vi "nanocal -- nuclear schottky fit V8.vi"() -> ()   [LabVIEW 2021] (continued)
\"mm1\" -> 0.000000000000   ,  \"mm2\" -> 0.000000000000   ,  \"mm3\" -> 0.000000000000   ,  \"T\" -> 0.300000000000   ,  \"B\" -> 2.000000000000   ,  \"θ\" -> 90.000000000000   ,  \"Reoff\" -> 0.000000000000   ,  \"Imoff\" -> 0.000000000000   ,  \"στ1\" -> 0.000000000000   ,  \"στS\" -> 0.000000000000   ,  \"στN\" -> 0.000000000000   ,  \"τ11 \" -> 0.000000000000   ,  \"τ12\" -> 0.000000000000   ,  \"τ22\" -> 0.000000000000   ,  \"τN1\" -> 0.000000000000   ,  \"τN2\" -> 0.000000000000   ,  \"σηlogτ1 \" -> 0.000000000000   ,  \"σηlogτS\" -> 0.000000000000   ,  \"σηlogτN\" -> 0.000000000000   ,  \"σlogτ1\" -> 0.000000000000   ,  \"σlogτS\" -> 0.000000000000   ,  \"σlogτN\" -> 0.000000000000   ,  \"σητ1\" -> 0.000000000000   ,  \"σητS \" -> 0.000000000000   ,  \"σητN\" -> 0.000000000000    |>   , \r\"IDS0584_220608_RAW_cal__ref_\" ->   <|    \"ζ\" -> 0.081243214747   ,  \"τ1\" -> 0.037135443189   ,  \"τS\" -> 0.014363776862   ,  \"τN\" -> 0.000724531165   ,  \"τC\" -> 0.001657389357   ,  \"κ0\" -> 0.000000001966   ,  \"mm1\" -> 0.000113270602   ,  \"mm2\" -> 0.016452146337   ,  \"mm3\" -> 0.038541546284   ,  \"T\" -> 0.360000000000   ,  \"B\" -> 2.000000000000   ,  \"θ\" -> 90.000000000000   ,  \"Reoff\" -> 0.000000000000   ,  \"Imoff\" -> 0.000000000000   ,  \"στ1\" -> 0.000570634052   ,  \"στS\" -> 0.000001716733   ,  \"στN\" -> 0.000008284109   ,  \"τ11 \" -> 0.000000000000   ,  \"τ12\" -> 0.000000000000   ,  \"τ22\" -> 0.000000000000   ,  \"τN1\" -> 0.000000000000   ,  \"τN2\" -> 0.000000000000   ,  \"σηlogτ1 \" -> 0.079922172346   ,  \"σηlogτS\" -> 0.000048378934   ,  \"σηlogτN\" -> 0.121081817682   ,  \"σlogτ1\" -> 0.015366291700   ,  \"σlogτS\" -> 0.000119518229   ,  \"σlogτN\" -> 0.011433750926   ,  \"σητ1\" -> 0.002967945291   ,  \"σητS \" -> 0.000000694904   ,  \"σητN\" -> 0.000087727550    |>   , \r\"IDS0584_220608_RAW_cal__sam_\" ->   <|    \"ζ\" -> 0.000000000000   ,  \"τ1\" -> 0.000000000000   ,  \"τS\" -> 0.000000000000   ,  \"τN\" -> 0.000000000000   ,  \"τC\" -> 0.000000000000   ,  \"κ0\" -> 0.000000000000   ,  \"mm1\" -> 0.000000000000   ,  \"mm2\" -> 0.000000000000   ,  \"mm3\" -> 0.000000000000   ,  \"T\" -> 0.360000000000   ,  \"B\" -> 2.000000000000   ,  \"θ\" -> 90.000000000000   ,  \"Reoff\" -> 0.000000000000   ,  \"Imoff\" -> 0.000000000000   ,  \"στ1\" -> 0.000000000000   ,  \"στS\" -> 0.000000000000   ,  \"στN\" -> 0.000000000000   ,  \"τ11 \" -> 0.000000000000   ,  \"τ12\" -> 0.000000000000   ,  \"τ22\" -> 0.000000000000   ,  \"τN1\" -> 0.000000000000   ,  \"τN2\" -> 0.000000000000   ,  \"σηlogτ1 \" -> 0.000000000000   ,  \"σηlogτS\" -> 0.000000000000   ,  \"σηlogτN\" -> 0.000000000000   ,  \"σlogτ1\" -> 0.000000000000   ,  \"σlogτS\" -> 0.000000000000   ,  \"σlogτN\" -> 0.000000000000   ,  \"σητ1\" -> 0.000000000000   ,  \"σητS \" -> 0.000000000000   ,  \"σητN\" -> 0.000000000000    |>   , \r\"IDS0585_220608_RAW_cal__ref_\" ->   <|    \"ζ\" -> 0.062678864922   ,  \"τ1\" -> 0.031193965489   ,  \"τS\" -> 0.014071158439   ,  \"τN\" -> 0.000589761795   ,  \"τC\" -> 0.002071432088   ,  \"κ0\" -> 0.000000002372   ,  \"mm1\" -> 0.000107994659   ,  \"mm2\" -> 0.016236809619   ,  \"mm3\" -> 0.032500443372   ,  \"T\" -> 0.420000000000   ,  \"B\" -> 2.000000000000   ,  \"θ\" -> 90.000000000000   ,  \"Reoff\" -> 0.000000000000   ,  \"Imoff\" -> 0.000000000000   ,  \"στ1\" -> 0.000397411460   ,  \"στS\" -> 0.000001349493   ,  \"στN\" -> 0.000005324437   ,  \"τ11 \" -> 0.000000000000   ,  \"τ12\" -> 0.000000000000   ,  \"τ22\" -> 0.000000000000   ,  \"τN1\" -> 0.000000000000   ,  \"τN2\" -> 0.000000000000   ,  \"σηlogτ1 \" -> 0.084702441661   ,  \"σηlogτS\" -> 0.000054291410   ,  \"σηlogτN\" -> 0.122395661985   ,  \"σlogτ1\" -> 0.012740010877   ,  \"σlogτS\" -> 0.000095904870   ,  \"σlogτN\" -> 0.009028114419   ,  \"σητ1\" -> 0.002642205042   ,  \"σητS \" -> 0.000000763943   ,  \"σητN\" -> 0.000072184285    |>   , \r\"IDS0585_220608_RAW_cal__sam_\" ->   <|    \"ζ\" -> 0.000000000000   ,  \"τ1\" -> 0.000000000000   ,  \"τS\" -> 0.000000000000   ,  \"τN\" -> 0.000000000000   ,  \"τC\" -> 0.000000000000   ,  \"κ0\" -> 0.000000000000   ,  \"mm1\" -> 0.000000000000   ,  \"mm2\" -> 0.000000000000   ,  \"mm3\" -> 0.000000000000   ,  \"T\" -> 0.420000000000   ,  \"B\" -> 2.000000000000   ,  \"θ\" -> 90.000000000000   ,  \"Reoff\" -> 0.000000000000   ,  \"Imoff\" -> 0.000000000000   ,  \"στ1\" -> 0.000000000000   ,  \"στS\" -> 0.000000000000   ,  \"στN\" -> 0.000000000000   ,  \"τ11 \" -> 0.000000000000   ,  \"τ12\" -> 0.000000000000   ,  \"τ22\" -> 0.000000000000   ,  \"τN1\" -> 0.000000000000   ,  \"τN2\" -> 0.000000000000   ,  \"σηlogτ1 \" -> 0.000000000000   ,  \"σηlogτS\" -> 0.000000000000   ,  \"σηlogτN\" -> 0.000000000000   ,  \"σlogτ1\" -> 0.000000000000   ,  \"σlogτS\" -> 0.000000000000   ,  \"σlogτN\" -> 0.000000000000   ,  \"σητ1\" -> 0.000000000000   ,  \"σητS \" -> 0.000000000000   ,  \"σητN\" -> 0.000000000000    |>   , \r\"IDS0586_220608_RAW_cal__ref_\" ->   <|    \"ζ\" -> 0.045613371440   ,  \"τ1\" -> 0.021724714281   ,  \"τS\" -> 0.014809258132   ,  \"τN\" -> 0.000242258752   ,  \"τC\" -> 0.002279252740   ,  \"κ0\" -> 0.000000003040   ,  \"mm1\" -> 0.000087097961   ,  \"mm2\" -> 0.016810935074   ,  \"mm3\" -> 0.022844001300   ,  \"T\" -> 0.520000000000   ,  \"B\" -> 2.000000000000   ,  \"θ\" -> 90.000000000000   ,  \"Reoff\" -> 0.000000000000   ,  \"Imoff\" -> 0.000000000000   ,  \"στ1\" -> 0.000379951004   ,  \"στS\" -> 0.000001062979   ,  \"στN\" -> 0.000002619514   ,  \"τ11 \" -> 0.000000000000   ,  \"τ12\" -> 0.000000000000   ,  \"τ22\" -> 0.000000000000   ,  \"τN1\" -> 0.000000000000   ,  \"τN2\" -> 0.000000000000   ,  \"σηlogτ1 \" -> 0.100214341065   ,  \"σηlogτS\" -> 0.000043367653   ,  \"σηlogτN\" -> 0.126292121784   ,  \"σlogτ1\" -> 0.017489344108   ,  \"σlogτS\" -> 0.000071778006   ,  \"σlogτN\" -> 0.010812876419   ,  \"σητ1\" -> 0.002177127926   ,  \"σητS \" -> 0.000000642243   ,  \"σητN\" -> 0.000030595372    |>   , \r\"IDS0586_220608_RAW_cal__sam_\" ->   <|    \"ζ\" -> 0.000000000000   ,  \"τ1\" -> 0.000000000000   ,  \"τS\" -> 0.000000000000   ,  \"τN\" -> 0.000000000000   ,  \"τC\" -> 0.000000000000   ,  \"κ0\" -> 0.000000000000   ,  \"mm1\" -> 0.000000000000   ,  \"mm2\" -> 0.000000000000   ,  \"mm3\" -> 0.000000000000   ,  \"T\" -> 0.520000000000   ,  \"B\" -> 2.000000000000   ,  \"θ\" -> 90.000000000000   ,  \"Reoff\" -> 0.000000000000   ,  \"Imoff\" -> 0.000000000000   ,  \"στ1\" -> 0.000000000000   ,  \"στS\" -> 0.000000000000   ,  \"στN\" -> 0.000000000000   ,  \"τ11 \" -> 0.000000000000   ,  \"τ12\" -> 0.000000000000   ,  \"τ22\" -> 0.000000000000   ,  \"τN1\" -> 0.000000000000   ,  \"τN2\" -> 0.000000000000   ,  \"σηlogτ1 \" -> 0.000000000000   ,  \"σηlogτS\" -> 0.000000000000   ,  \"σηlogτN\" -> 0.000000000000   ,  \"σlogτ1\" -> 0.000000000000   ,  \"σlogτS\" -> 0.000000000000   ,  \"σlogτN\" -> 0.000000000000   ,  \"σητ1\" -> 0.000000000000   ,  \"σητS \" -> 0.000000000000   ,  \"σητN\" -> 0.000000000000    |>   , \r\"IDS0587_220608_RAW_cal__ref_\" ->   <|    \"ζ\" -> 0.037305312817   ,  \"τ1\" -> 0.022015385532   ,  \"τS\" -> 0.015983002513   ,  \"τN\" -> 0.000140757523   ,  \"τC\" -> 0.002926821930   ,  \"κ0\" -> 0.000000003719   ,  \"mm1\" -> 0.000089879141   ,  \"mm2\" -> 0.018616997914   ,  \"mm3\" -> 0.022960592355   ,  \"T\" -> 0.620000000000   ,  \"B\" -> 2.000000000000   ,  \"θ\" -> 90.000000000000   ,  \"Reoff\" -> 0.000000000000   ,  \"Imoff\" -> 0.000000000000   ,  \"στ1\" -> 0.001387023615   ,  \"στS\" -> 0.000002362873   ,  \"στN\" -> 0.000005327242   ,  \"τ11 \" -> 0.000000000000   ,  \"τ12\" -> 0.000000000000   ,  \"τ22\" -> 0.000000000000   ,  \"τN1\" -> 0.000000000000   ,  \"τN2\" -> 0.000000000000   ,  \"σηlogτ1 \" -> 0.104062754618   ,  \"σηlogτS\" -> 0.000026827334   ,  \"σηlogτN\" -> 0.127171087311   ,  \"σlogτ1\" -> 0.063002467668   ,  \"σlogτS\" -> 0.000147836639   ,  \"σlogτN\" -> 0.037846942559   ,  \"σητ1\" -> 0.002290981662   ,  \"σητS \" -> 0.000000428781   ,  \"σητN\" -> 0.000017900287    |>   , \r\"IDS0587_220608_RAW_cal__sam_\" ->   <|    \"ζ\" -> 0.000000000000   ,  \"τ1\" -> 0.000000000000   ,  \"τS\" -> 0.000000000000   ,  \"τN\" -> 0.000000000000   ,  \"τC\" -> 0.000000000000   ,  \"κ0\" -> 0.000000000000   ,  \"mm1\" -> 0.000000000000   ,  \"mm2\" -> 0.000000000000   ,  \"mm3\" -> 0.000000000000   ,  \"T\" -> 0.620000000000   ,  \"B\" -> 2.000000000000   ,  \"θ\" -> 90.000000000000   ,  \"Reoff\" -> 0.000000000000   ,  \"Imoff\" -> 0.000000000000   ,  \"στ1\" -> 0.000000000000   ,  \"στS\" -> 0.000000000000   ,  \"στN\" -> 0.000000000000   ,  \"τ11 \" -> 0.000000000000   ,  \"τ12\" -> 0.000000000000   ,  \"τ22\" -> 0.000000000000   ,  \"τN1\" -> 0.000000000000   ,  \"τN2\" -> 0.000000000000   ,  \"σηlogτ1 \" -> 0.000000000000   ,  \"σηlogτS\" -> 0.000000000000   ,  \"σηlogτN\" -> 0.000000000000   ,  \"σlogτ1\" -> 0.000000000000   ,  \"σlogτS\" -> 0.000000000000   ,  \"σlogτN\" -> 0.000000000000   ,  \"σητ1\" -> 0.000000000000   ,  \"σητS \" -> 0.000000000000   ,  \"σητN\" -> 0.000000000000    |>   , \r\"IDS0588_220608_RAW_cal__ref_\" ->   <|    \"ζ\" -> 0.025909739103   ,  \"τ1\" -> 0.011339568662   ,  \"τS\" -> 0.019465034891   ,  \"τN\" -> 0.000064248096   ,  \"τC\" -> 0.003634951458   ,  \"κ0\" -> 0.000000005097   ,  \"mm1\" -> 0.000077921965   ,  \"mm2\" -> 0.011278943418   ,  \"mm3\" -> 0.023652936351   ,  \"T\" -> 0.820000000000   ,  \"B\" -> 2.000000000000   ,  \"θ\" -> 90.000000000000   ,  \"Reoff\" -> 0.000000000000   ,  \"Imoff\" -> 0.000000000000   ,  \"στ1\" -> 0.000804918682   ,  \"στS\" -> 0.000001968832   ,  \"στN\" -> 0.000002244062   ,  \"τ11 \" -> 0.000000000000   ,  \"τ12\" -> 0.000000000000   ,  \"τ22\" -> 0.000000000000   ,  \"τN1\" -> 0.000000000000   ,  \"τN2\" -> 0.000000000000   ,  \"σηlogτ1 \" -> 0.166612292303   ,  \"σηlogτS\" -> 0.000038744835   ,  \"σηlogτN\" -> 0.138837522658   ,  \"σlogτ1\" -> 0.070983183376   ,  \"σlogτS\" -> 0.000101147100   ,  \"σlogτN\" -> 0.034928067640   ,  \"σητ1\" -> 0.001889311528   ,  \"σητS \" -> 0.000000754170   ,  \"σητN\" -> 0.000008920046    |>   , \r\"IDS0588_220608_RAW_cal__sam_\" ->   <|    \"ζ\" -> 0.000000000000   ,  \"τ1\" -> 0.000000000000   ,  \"τS\" -> 0.000000000000   ,  \"τN\" -> 0.000000000000   ,  \"τC\" -> 0.000000000000   ,  \"κ0\" -> 0.000000000000   ,  \"mm1\" -> 0.000000000000   ,  \"mm2\" -> 0.000000000000   ,  \"mm3\" -> 0.000000000000   ,  \"T\" -> 0.820000000000   ,  \"B\" -> 2.000000000000   ,  \"θ\" -> 90.000000000000   ,  \"Reoff\" -> 0.000000000000   ,  \"Imoff\" -> 0.000000000000   ,  \"στ1\" -> 0.000000000000   ,  \"στS\" -> 0.000000000000   ,  \"στN\" -> 0.000000000000   ,  \"τ11 \" -> 0.000000000000   ,  \"τ12\" -> 0.000000000000   ,  \"τ22\" -> 0.000000000000   ,  \"τN1\" -> 0.000000000000   ,  \"τN2\" -> 0.000000000000   ,  \"σηlogτ1 \" -> 0.000000000000   ,  \"σηlogτS\" -> 0.000000000000   ,  \"σηlogτN\" -> 0.000000000000   ,  \"σlogτ1\" -> 0.000000000000   ,  \"σlogτS\" -> 0.000000000000   ,  \"σlogτN\" -> 0.000000000000   ,  \"σητ1\" -> 0.000000000000   ,  \"σητS \" -> 0.000000000000   ,  \"σητN\" -> 0.000000000000    |>   , \r\"IDS0589_220608_RAW_cal__ref_\" ->   <|    \"ζ\" -> 0.019947361770   ,  \"τ1\" -> 0.011361864478   ,  \"τS\" -> 0.027583078448   ,  \"τN\" -> 0.000020419433   ,  \"τC\" -> 0.003703000671   ,  \"κ0\" -> 0.000000007195   ,  \"mm1\" -> 0.000064126126   ,  \"mm2\" -> 0.011350297657   ,  \"mm3\" -> 0.031804556205   ,  \"T\" -> 1.120000000000   ,  \"B\" -> 2.000000000000   ,  \"θ\" -> 90.000000000000   ,  \"Reoff\" -> 0.000000000000   ,  \"Imoff\" -> 0.000000000000   ,  \"στ1\" -> 0.003857512169   ,  \"στS\" -> 0.000003346779   ,  \"στN\" -> 0.000003441616   ,  \"τ11 \" -> 0.000000000000   ,  \"τ12\" -> 0.000000000000   ,  \"τ22\" -> 0.000000000000   ,  \"τN1\" -> 0.000000000000   ,  \"τN2\" -> 0.000000000000   ,  \"σηlogτ1 \" -> 0.199481573795   ,  \"σηlogτS\" -> 0.000012934123   ,  \"σηlogτN\" -> 0.143434929162   ,  \"σlogτ1\" -> 0.339514009879   ,  \"σlogτS\" -> 0.000121334492   ,  \"σlogτN\" -> 0.168546132727   ,  \"σητ1\" -> 0.002266482607   ,  \"σητS \" -> 0.000000356763   ,  \"σητN\" -> 0.000002928860    |>   , \r\"IDS0589_220608_RAW_cal__sam_\" ->   <|    \"ζ\" -> 0.000000000000   ,  \"τ1\" -> 0.000000000000   ,  \"τS\" -> 0.000000000000   ,  \"τN\" -> 0.000000000000   ,  \"τC\" -> 0.000000000000   ,  \"κ0\" -> 0.000000000000   ,  \"mm1\" -> 0.000000000000   ,  \"mm2\" -> 0.000000000000   ,  \"mm3\" -> 0.000000000000   ,  \"T\" -> 1.120000000000   ,  \"B\" -> 2.000000000000   ,  \"θ\" -> 90.000000000000   ,  \"Reoff\" -> 0.000000000000   ,  \"Imoff\" -> 0.000000000000   ,  \"στ1\" -> 0.000000000000   ,  \"στS\" -> 0.000000000000   ,  \"στN\" -> 0.000000000000   ,  \"τ11 \" -> 0.000000000000   ,  \"τ12\" -> 0.000000000000   ,  \"τ22\" -> 0.000000000000   ,  \"τN1\" -> 0.000000000000   ,  \"τN2\" -> 0.000000000000   ,  \"σηlogτ1 \" -> 0.000000000000   ,  \"σηlogτS\" -> 0.000000000000   ,  \"σηlogτN\" -> 0.000000000000   ,  \"σlogτ1\" -> 0.000000000000   ,  \"σlogτS\" -> 0.000000000000   ,  \"σlogτN\" -> 0.000000000000   ,  \"σητ1\" -> 0.000000000000   ,  \"σητS \" -> 0.000000000000   ,  \"σητN\" -> 0.000000000000    |>   , \r\"IDS0590_220608_RAW_cal__ref_\" ->   <|    \"ζ\" -> 0.015986824181   ,  \"τ1\" -> 0.008744331225   ,  \"τS\" -> 0.042647705878   ,  \"τN\" -> 0.000007777315   ,  \"τC\" -> 0.003875042779   ,  \"κ0\" -> 0.000000010497   ,  \"mm1\" -> 0.000056035896   ,  \"mm2\" -> 0.008742533558   ,  \"mm3\" -> 0.047158213453   ,  \"T\" -> 1.600000000000   ,  \"B\" -> 2.000000000000   ,  \"θ\" -> 90.000000000000   ,  \"Reoff\" -> 0.000000000000   ,  \"Imoff\" -> 0.000000000000   ,  \"στ1\" -> 0.012923457313   ,  \"στS\" -> 0.000006598601   ,  \"στN\" -> 0.000006323440   ,  \"τ11 \" -> 0.000000000000   ,  \"τ12\" -> 0.000000000000   ,  \"τ22\" -> 0.000000000000   ,  \"τN1\" -> 0.000000000000   ,  \"τN2\" -> 0.000000000000   ,  \"σηlogτ1 \" -> 0.292115286414   ,  \"σηlogτS\" -> 0.000006686874   ,  \"σηlogτN\" -> 0.152613381435   ,  \"σlogτ1\" -> 1.477924038063   ,  \"σlogτS\" -> 0.000154723460   ,  \"σlogτN\" -> 0.813062124380   ,  \"σητ1\" -> 0.002554352820   ,  \"σητS \" -> 0.000000285180   ,  \"σητN\" -> 0.000001186922    |>   , \r\"IDS0590_220608_RAW_cal__sam_\" ->   <|    \"ζ\" -> 0.000000000000   ,  \"τ1\" -> 0.000000000000   ,  \"τS\" -> 0.000000000000   ,  \"τN\" -> 0.000000000000   ,  \"τC\" -> 0.000000000000   ,  \"κ0\" -> 0.000000000000   ,  \"mm1\" -> 0.000000000000   ,  \"mm2\" -> 0.000000000000   ,  \"mm3\" -> 0.000000000000   ,  \"T\" -> 1.600000000000   ,  \"B\" -> 2.000000000000   ,  \"θ\" -> 90.000000000000   ,  \"Reoff\" -> 0.000000000000   ,  \"Imoff\" -> 0.000000000000   ,  \"στ1\" -> 0.000000000000   ,  \"στS\" -> 0.000000000000   ,  \"στN\" -> 0.000000000000   ,  \"τ11 \" -> 0.000000000000   ,  \"τ12\" -> 0.000000000000   ,  \"τ22\" -> 0.000000000000   ,  \"τN1\" -> 0.000000000000   ,  \"τN2\" -> 0.000000000000   ,  \"σηlogτ1 \" -> 0.000000000000   ,  \"σηlogτS\" -> 0.000000000000   ,  \"σηlogτN\" -> 0.000000000000   ,  \"σlogτ1\" -> 0.000000000000   ,  \"σlogτS\" -> 0.000000000000   ,  \"σlogτN\" -> 0.000000000000   ,  \"σητ1\" -> 0.000000000000   ,  \"σητS \" -> 0.000000000000   ,  \"σητN\" -> 0.000000000000    |>   , \r\"IDS0591_220608_RAW_cal__ref_\" ->   <|    \"ζ\" -> 0.017496232400   ,  \"τ1\" -> 0.009379616300   ,  \"τS\" -> 0.011529506794   ,  \"τN\" -> 0.000002471799   ,  \"τC\" -> 0.003013860200   ,  \"κ0\" -> 0.000000015619   ,  \"mm1\" -> 0.000041347609   ,  \"mm2\" -> 0.009375196223   ,  \"mm3\" -> 0.014710677438   ,  \"T\" -> 2.300000000000   ,  \"B\" -> 2.000000000000   ,  \"θ\" -> 90.000000000000   ,  \"Reoff\" -> 0.000000000000   ,  \"Imoff\" -> 0.000000000000   ,  \"στ1\" -> 0.011594693378   ,  \"στS\" -> 0.000001156302   ,  \"στN\" -> 0.000001553870   ,  \"τ11 \" -> 0.000000000000   ,  \"τ12\" -> 0.000000000000   ,  \"τ22\" -> 0.000000000000   ,  \"τN1\" -> 0.000000000000   ,  \"τN2\" -> 0.000000000000   ,  \"σηlogτ1 \" -> 0.141137332089   ,  \"σηlogτS\" -> 0.000001654332   ,  \"σηlogτN\" -> 0.134661811699   ,  \"σlogτ1\" -> 1.236158602592   ,  \"σlogτS\" -> 0.000100290701   ,  \"σlogτN\" -> 0.628639383488   ,  \"σητ1\" -> 0.001323814021   ,  \"σητS \" -> 0.000000019074   ,  \"σητN\" -> 0.000000332857    |>   , \r\"IDS0591_220608_RAW_cal__sam_\" ->   <|    \"ζ\" -> 0.000000000000   ,  \"τ1\" -> 0.000000000000   ,  \"τS\" -> 0.000000000000   ,  \"τN\" -> 0.000000000000   ,  \"τC\" -> 0.000000000000   ,  \"κ0\" -> 0.000000000000   ,  \"mm1\" -> 0.000000000000   ,  \"mm2\" -> 0.000000000000   ,  \"mm3\" -> 0.000000000000   ,  \"T\" -> 2.300000000000   ,  \"B\" -> 2.000000000000   ,  \"θ\" -> 90.000000000000   ,  \"Reoff\" -> 0.000000000000   ,  \"Imoff\" -> 0.000000000000   ,  \"στ1\" -> 0.000000000000   ,  \"στS\" -> 0.000000000000   ,  \"στN\" -> 0.000000000000   ,  \"τ11 \" -> 0.000000000000   ,  \"τ12\" -> 0.000000000000   ,  \"τ22\" -> 0.000000000000   ,  \"τN1\" -> 0.000000000000   ,  \"τN2\" -> 0.000000000000   ,  \"σηlogτ1 \" -> 0.000000000000   ,  \"σηlogτS\" -> 0.000000000000   ,  \"σηlogτN\" -> 0.000000000000   ,  \"σlogτ1\" -> 0.000000000000   ,  \"σlogτS\" -> 0.000000000000   ,  \"σlogτN\" -> 0.000000000000   ,  \"σητ1\" -> 0.000000000000   ,  \"σητS \" -> 0.000000000000   ,  \"σητN\" -> 0.000000000000    |>   , \r\"IDS0592_220608_RAW_cal__ref_\" ->   <|    \"ζ\" -> 0.019029594007   ,  \"τ1\" -> 0.017581938574   ,  \"τS\" -> 0.009721936381   ,  \"τN\" -> 0.000001128241   ,  \"τC\" -> 0.002339976361   ,  \"κ0\" -> 0.000000022398   ,  \"mm1\" -> 0.000035450791   ,  \"mm2\" -> 0.012208855819   ,  \"mm3\" -> 0.017585698919   ,  \"T\" -> 3.100000000000   ,  \"B\" -> 2.000000000000   ,  \"θ\" -> 90.000000000000   ,  \"Reoff\" -> 0.000000000000   ,  \"Imoff\" -> 0.000000000000   ,  \"στ1\" -> 0.049820756354   ,  \"στS\" -> 0.000000710276   ,  \"στN\" -> 0.000002087356   ,  \"τ11 \" -> 0.000000000000   ,  \"τ12\" -> 0.000000000000   ,  \"τ22\" -> 0.000000000000   ,  \"τN1\" -> 0.000000000000   ,  \"τN2\" -> 0.000000000000   ,  \"σηlogτ1 \" -> 0.093372347104   ,  \"σηlogτS\" -> 0.000000231794   ,  \"σηlogτN\" -> 0.124583503268   ,  \"σlogτ1\" -> 2.833632716014   ,  \"σlogτS\" -> 0.000073059076   ,  \"σlogτN\" -> 1.850098255960   ,  \"σητ1\" -> 0.001641666871   ,  \"σητS \" -> 0.000000002253   ,  \"σητN\" -> 0.000000140560    |>   , \r\"IDS0592_220608_RAW_cal__sam_\" ->   <|    \"ζ\" -> 0.000000000000   ,  \"τ1\" -> 0.000000000000   ,  \"τS\" -> 0.000000000000   ,  \"τN\" -> 0.000000000000   ,  \"τC\" -> 0.000000000000   ,  \"κ0\" -> 0.000000000000   ,  \"mm1\" -> 0.000000000000   ,  \"mm2\" -> 0.000000000000   ,  \"mm3\" -> 0.000000000000   ,  \"T\" -> 3.100000000000   ,  \"B\" -> 2.000000000000   ,  \"θ\" -> 90.000000000000   ,  \"Reoff\" -> 0.000000000000   ,  \"Imoff\" -> 0.000000000000   ,  \"στ1\" -> 0.000000000000   ,  \"στS\" -> 0.000000000000   ,  \"στN\" -> 0.000000000000   ,  \"τ11 \" -> 0.000000000000   ,  \"τ12\" -> 0.000000000000   ,  \"τ22\" -> 0.000000000000   ,  \"τN1\" -> 0.000000000000   ,  \"τN2\" -> 0.000000000000   ,  \"σηlogτ1 \" -> 0.000000000000   ,  \"σηlogτS\" -> 0.000000000000   ,  \"σηlogτN\" -> 0.000000000000   ,  \"σlogτ1\" -> 0.000000000000   ,  \"σlogτS\" -> 0.000000000000   ,  \"σlogτN\" -> 0.000000000000   ,  \"σητ1\" -> 0.000000000000   ,  \"σητS \" -> 0.000000000000   ,  \"σητN\" -> 0.000000000000    |>   , \r\"IDS0593_220608_RAW_cal__ref_\" ->   <|    \"ζ\" -> 0.021294906614   ,  \"τ1\" -> 0.016155792293   ,  \"τS\" -> 0.006010538470   ,  \"τN\" -> 0.000000265204   ,  \"τC\" -> 0.001740380936   ,  \"κ0\" -> 0.000000055295   ,  \"mm1\" -> 0.000028374877   ,  \"mm2\" -> 0.007850282637   ,  \"mm3\" -> 0.016156318892   ,  \"T\" -> 5.700000000000   ,  \"B\" -> 2.000000000000   ,  \"θ\" -> 90.000000000000   ,  \"Reoff\" -> 0.000000000000   ,  \"Imoff\" -> 0.000000000000   ,  \"στ1\" -> 0.179781175728   ,  \"στS\" -> 0.000000482130   ,  \"στN\" -> 0.000002158391   ,  \"τ11 \" -> 0.000000000000   ,  \"τ12\" -> 0.000000000000   ,  \"τ22\" -> 0.000000000000   ,  \"τN1\" -> 0.000000000000   ,  \"τN2\" -> 0.000000000000   ,  \"σηlogτ1 \" -> 0.081363569031   ,  \"σηlogτS\" -> 0.000000046538   ,  \"σηlogτN\" -> 0.121425477475   ,  \"σlogτ1\" -> 11.127970233063   ,  \"σlogτS\" -> 0.000080214100   ,  \"σlogτN\" -> 8.138592608049   ,  \"σητ1\" -> 0.001314492921   ,  \"σητS \" -> 0.000000000280   ,  \"σητN\" -> 0.000000032203    |>   , \r\"IDS0593_220608_RAW_cal__sam_\" ->   <|    \"ζ\" -> 0.000000000000   ,  \"τ1\" -> 0.000000000000   ,  \"τS\" -> 0.000000000000   ,  \"τN\" -> 0.000000000000   ,  \"τC\" -> 0.000000000000   ,  \"κ0\" -> 0.000000000000   ,  \"mm1\" -> 0.000000000000   ,  \"mm2\" -> 0.000000000000   ,  \"mm3\" -> 0.000000000000   ,  \"T\" -> 5.700000000000   ,  \"B\" -> 2.000000000000   ,  \"θ\" -> 90.000000000000   ,  \"Reoff\" -> 0.000000000000   ,  \"Imoff\" -> 0.000000000000   ,  \"στ1\" -> 0.000000000000   ,  \"στS\" -> 0.000000000000   ,  \"στN\" -> 0.000000000000   ,  \"τ11 \" -> 0.000000000000   ,  \"τ12\" -> 0.000000000000   ,  \"τ22\" -> 0.000000000000   ,  \"τN1\" -> 0.000000000000   ,  \"τN2\" -> 0.000000000000   ,  \"σηlogτ1 \" -> 0.000000000000   ,  \"σηlogτS\" -> 0.000000000000   ,  \"σηlogτN\" -> 0.000000000000   ,  \"σlogτ1\" -> 0.000000000000   ,  \"σlogτS\" -> 0.000000000000   ,  \"σlogτN\" -> 0.000000000000   ,  \"σητ1\" -> 0.000000000000   ,  \"σητS \" -> 0.000000000000   ,  \"σητN\" -> 0.000000000000    |>   , \r\"IDS0595_220608_RAW_cal__ref_\" ->   <|    \"ζ\" -> 0.244875688813   ,  \"τ1\" -> 0.040857302003   ,  \"τS\" -> 0.046628683614   ,  \"τN\" -> 0.009593794520   ,  \"τC\" -> 0.000917891247   ,  \"κ0\" -> 0.000000000890   ,  \"mm1\" -> 0.000178281936   ,  \"mm2\" -> 0.029128430859   ,  \"mm3\" -> 0.082458476649   ,  \"T\" -> 0.200000000000   ,  \"B\" -> 4.000000000000   ,  \"θ\" -> 90.000000000000   ,  \"Reoff\" -> 0.000000000000   ,  \"Imoff\" -> 0.000000000000   ,  \"στ1\" -> 0.000204250954   ,  \"στS\" -> 0.000016140182   ,  \"στN\" -> 0.000025700358   ,  \"τ11 \" -> 0.000000000000   ,  \"τ12\" -> 0.000000000000   ,  \"τ22\" -> 0.000000000000   ,  \"τN1\" -> 0.000000000000   ,  \"τN2\" -> 0.000000000000   ,  \"σηlogτ1 \" -> 0.133588413120   ,  \"σηlogτS\" -> 0.001269402003   ,  \"σηlogτN\" -> 0.135197574519   ,  \"σlogτ1\" -> 0.004999129754   ,  \"σlogτS\" -> 0.000346142779   ,  \"σlogτN\" -> 0.002678852216   ,  \"σητ1\" -> 0.005458062139   ,  \"σητS \" -> 0.000059190544   ,  \"σητN\" -> 0.001297057749    |>   , \r\"IDS0595_220608_RAW_cal__sam_\" ->   <|    \"ζ\" -> 0.000000000000   ,  \"τ1\" -> 0.000000000000   ,  \"τS\" -> 0.000000000000   ,  \"τN\" -> 0.000000000000   ,  \"τC\" -> 0.000000000000   ,  \"κ0\" -> 0.000000000000   ,  \"mm1\" -> 0.000000000000   ,  \"mm2\" -> 0.000000000000   ,  \"mm3\" -> 0.000000000000   ,  \"T\" -> 0.200000000000   ,  \"B\" -> 4.000000000000   ,  \"θ\" -> 90.000000000000   ,  \"Reoff\" -> 0.000000000000   ,  \"Imoff\" -> 0.000000000000   ,  \"στ1\" -> 0.000000000000   ,  \"στS\" -> 0.000000000000   ,  \"στN\" -> 0.000000000000   ,  \"τ11 \" -> 0.000000000000   ,  \"τ12\" -> 0.000000000000   ,  \"τ22\" -> 0.000000000000   ,  \"τN1\" -> 0.000000000000   ,  \"τN2\" -> 0.000000000000   ,  \"σηlogτ1 \" -> 0.000000000000   ,  \"σηlogτS\" -> 0.000000000000   ,  \"σηlogτN\" -> 0.000000000000   ,  \"σlogτ1\" -> 0.000000000000   ,  \"σlogτS\" -> 0.000000000000   ,  \"σlogτN\" -> 0.000000000000   ,  \"σητ1\" -> 0.000000000000   ,  \"σητS \" -> 0.000000000000   ,  \"σητN\" -> 0.000000000000    |>   , \r\"IDS0596_220608_RAW_cal__ref_\" ->   <|    \"ζ\" -> 0.344647843466   ,  \"τ1\" -> 0.055962851231   ,  \"τS\" -> 0.054806527829   ,  \"τN\" -> 0.019330510227   ,  \"τC\" -> 0.000846071488   ,  \"κ0\" -> 0.000000000723   ,  \"mm1\" -> 0.000215013630   ,  \"mm2\" -> 0.034022445863   ,  \"mm3\" -> 0.122259671569   ,  \"T\" -> 0.170000000000   ,  \"B\" -> 4.000000000000   ,  \"θ\" -> 90.000000000000   ,  \"Reoff\" -> 0.000000000000   ,  \"Imoff\" -> 0.000000000000   ,  \"στ1\" -> 0.000271742026   ,  \"στS\" -> 0.000028779791   ,  \"στN\" -> 0.000052361049   ,  \"τ11 \" -> 0.000000000000   ,  \"τ12\" -> 0.000000000000   ,  \"τ22\" -> 0.000000000000   ,  \"τN1\" -> 0.000000000000   ,  \"τN2\" -> 0.000000000000   ,  \"σηlogτ1 \" -> 0.127696466200   ,  \"σηlogτS\" -> 0.001816681804   ,  \"σηlogτN\" -> 0.135107921466   ,  \"σlogτ1\" -> 0.004855757346   ,  \"σlogτS\" -> 0.000525116114   ,  \"σlogτN\" -> 0.002708725676   ,  \"σητ1\" -> 0.007146258341   ,  \"σητS \" -> 0.000099566022   ,  \"σητN\" -> 0.002611705058    |>   , \r\"IDS0596_220608_RAW_cal__sam_\" ->   <|    \"ζ\" -> 0.000000000000   ,  \"τ1\" -> 0.000000000000   ,  \"τS\" -> 0.000000000000   ,  \"τN\" -> 0.000000000000   ,  \"τC\" -> 0.000000000000   ,  \"κ0\" -> 0.000000000000   ,  \"mm1\" -> 0.000000000000   ,  \"mm2\" -> 0.000000000000   ,  \"mm3\" -> 0.000000000000   ,  \"T\" -> 0.170000000000   ,  \"B\" -> 4.000000000000   ,  \"θ\" -> 90.000000000000   ,  \"Reoff\" -> 0.000000000000   ,  \"Imoff\" -> 0.000000000000   ,  \"στ1\" -> 0.000000000000   ,  \"στS\" -> 0.000000000000   ,  \"στN\" -> 0.000000000000   ,  \"τ11 \" -> 0.000000000000   ,  \"τ12\" -> 0.000000000000   ,  \"τ22\" -> 0.000000000000   ,  \"τN1\" -> 0.000000000000   ,  \"τN2\" -> 0.000000000000   ,  \"σηlogτ1 \" -> 0.000000000000   ,  \"σηlogτS\" -> 0.000000000000   ,  \"σηlogτN\" -> 0.000000000000   ,  \"σlogτ1\" -> 0.000000000000   ,  \"σlogτS\" -> 0.000000000000   ,  \"σlogτN\" -> 0.000000000000   ,  \"σητ1\" -> 0.000000000000   ,  \"σητS \" -> 0.000000000000   ,  \"σητN\" -> 0.000000000000    |>   , \r\"IDS0597_220608_RAW_cal__ref_\" ->   <|    \"ζ\" -> 0.438135386554   ,  \"τ1\" -> 0.068308117245   ,  \"τS\" -> 0.065117760308   ,  \"τN\" -> 0.029655865549   ,  \"τC\" -> 0.000827290289   ,  \"κ0\" -> 0.000000000603   ,  \"mm1\" -> 0.000250492842   ,  \"mm2\" -> 0.038649413418   ,  \"mm3\" -> 0.166532806331   ,  \"T\" -> 0.150000000000   ,  \"B\" -> 4.000000000000   ,  \"θ\" -> 90.000000000000   ,  \"Reoff\" -> 0.000000000000   ,  \"Imoff\" -> 0.000000000000   ,  \"στ1\" -> 0.000386864233   ,  \"στS\" -> 0.000050730025   ,  \"στN\" -> 0.000093978346   ,  \"τ11 \" -> 0.000000000000   ,  \"τ12\" -> 0.000000000000   ,  \"τ22\" -> 0.000000000000   ,  \"τN1\" -> 0.000000000000   ,  \"τN2\" -> 0.000000000000   ,  \"σηlogτ1 \" -> 0.130185307771   ,  \"σηlogτS\" -> 0.002377860764   ,  \"σηlogτN\" -> 0.136705910950   ,  \"σlogτ1\" -> 0.005663517726   ,  \"σlogτS\" -> 0.000779050517   ,  \"σlogτN\" -> 0.003168963187   ,  \"σητ1\" -> 0.008892713267   ,  \"σητS \" -> 0.000154840967   ,  \"σητN\" -> 0.004054132115    |>   , \r\"IDS0597_220608_RAW_cal__sam_\" ->   <|    \"ζ\" -> 0.000000000000   ,  \"τ1\" -> 0.000000000000   ,  \"τS\" -> 0.000000000000   ,  \"τN\" -> 0.000000000000   ,  \"τC\" -> 0.000000000000   ,  \"κ0\" -> 0.000000000000   ,  \"mm1\" -> 0.000000000000   ,  \"mm2\" -> 0.000000000000   ,  \"mm3\" -> 0.000000000000   ,  \"T\" -> 0.150000000000   ,  \"B\" -> 4.000000000000   ,  \"θ\" -> 90.000000000000   ,  \"Reoff\" -> 0.000000000000   ,  \"Imoff\" -> 0.000000000000   ,  \"στ1\" -> 0.000000000000   ,  \"στS\" -> 0.000000000000   ,  \"στN\" -> 0.000000000000   ,  \"τ11 \" -> 0.000000000000   ,  \"τ12\" -> 0.000000000000   ,  \"τ22\" -> 0.000000000000   ,  \"τN1\" -> 0.000000000000   ,  \"τN2\" -> 0.000000000000   ,  \"σηlogτ1 \" -> 0.000000000000   ,  \"σηlogτS\" -> 0.000000000000   ,  \"σηlogτN\" -> 0.000000000000   ,  \"σlogτ1\" -> 0.000000000000   ,  \"σlogτS\" -> 0.000000000000   ,  \"σlogτN\" -> 0.000000000000   ,  \"σητ1\" -> 0.000000000000   ,  \"σητS \" -> 0.000000000000   ,  \"σητN\" -> 0.000000000000    |>   , \r\"IDS0598_220609_RAW_cal__ref_\" ->   <|    \"ζ\" -> 0.657739242664   ,  \"τ1\" -> 0.094390866023   ,  \"τS\" -> 0.092485939026   ,  \"τN\" -> 0.075235660574   ,  \"τC\" -> 0.000808280402   ,  \"κ0\" -> 0.000000000441   ,  \"mm1\" -> 0.000319678865   ,  \"mm2\" -> 0.044160231701   ,  \"mm3\" -> 0.328757913358   ,  \"T\" -> 0.120000000000   ,  \"B\" -> 4.000000000000   ,  \"θ\" -> 90.000000000000   ,  \"Reoff\" -> 0.000000000000   ,  \"Imoff\" -> 0.000000000000   ,  \"στ1\" -> 0.000620717106   ,  \"στS\" -> 0.000143661942   ,  \"στN\" -> 0.000275186110   ,  \"τ11 \" -> 0.000000000000   ,  \"τ12\" -> 0.000000000000   ,  \"τ22\" -> 0.000000000000   ,  \"τN1\" -> 0.000000000000   ,  \"τN2\" -> 0.000000000000   ,  \"σηlogτ1 \" -> 0.141859959037   ,  \"σηlogτS\" -> 0.004605254266   ,  \"σηlogτN\" -> 0.143938852633   ,  \"σlogτ1\" -> 0.006576029356   ,  \"σlogτS\" -> 0.001553338196   ,  \"σlogτN\" -> 0.003657655270   ,  \"σητ1\" -> 0.013390284387   ,  \"σητS \" -> 0.000425921265   ,  \"σητN\" -> 0.010829334660    |>   , \r\"IDS0598_220609_RAW_cal__sam_\" ->   <|    \"ζ\" -> 0.000000000000   ,  \"τ1\" -> 0.000000000000   ,  \"τS\" -> 0.000000000000   ,  \"τN\" -> 0.000000000000   ,  \"τC\" -> 0.000000000000   ,  \"κ0\" -> 0.000000000000   ,  \"mm1\" -> 0.000000000000   ,  \"mm2\" -> 0.000000000000   ,  \"mm3\" -> 0.000000000000   ,  \"T\" -> 0.120000000000   ,  \"B\" -> 4.000000000000   ,  \"θ\" -> 90.000000000000   ,  \"Reoff\" -> 0.000000000000   ,  \"Imoff\" -> 0.000000000000   ,  \"στ1\" -> 0.000000000000   ,  \"στS\" -> 0.000000000000   ,  \"στN\" -> 0.000000000000   ,  \"τ11 \" -> 0.000000000000   ,  \"τ12\" -> 0.000000000000   ,  \"τ22\" -> 0.000000000000   ,  \"τN1\" -> 0.000000000000   ,  \"τN2\" -> 0.000000000000   ,  \"σηlogτ1 \" -> 0.000000000000   ,  \"σηlogτS\" -> 0.000000000000   ,  \"σηlogτN\" -> 0.000000000000   ,  \"σlogτ1\" -> 0.000000000000   ,  \"σlogτS\" -> 0.000000000000   ,  \"σlogτN\" -> 0.000000000000   ,  \"σητ1\" -> 0.000000000000   ,  \"σητS \" -> 0.000000000000   ,  \"σητN\" -> 0.000000000000    |>   , \r\"IDS0599_220609_RAW_cal__ref_\" ->   <|    \"ζ\" -> 0.160640867986   ,  \"τ1\" -> 0.030730944542   ,  \"τS\" -> 0.038747882734   ,  \"τN\" -> 0.003719905451   ,  \"τC\" -> 0.000979240032   ,  \"κ0\" -> 0.000000001232   ,  \"mm1\" -> 0.000133029555   ,  \"mm2\" -> 0.025373328786   ,  \"mm3\" -> 0.055493676773   ,  \"T\" -> 0.250000000000   ,  \"B\" -> 4.000000000000   ,  \"θ\" -> 90.000000000000   ,  \"Reoff\" -> 0.000000000000   ,  \"Imoff\" -> 0.000000000000   ,  \"στ1\" -> 0.000234620158   ,  \"στS\" -> 0.000010118580   ,  \"στN\" -> 0.000014838249   ,  \"τ11 \" -> 0.000000000000   ,  \"τ12\" -> 0.000000000000   ,  \"τ22\" -> 0.000000000000   ,  \"τN1\" -> 0.000000000000   ,  \"τN2\" -> 0.000000000000   ,  \"σηlogτ1 \" -> 0.136644624286   ,  \"σηlogτS\" -> 0.000655650020   ,  \"σηlogτN\" -> 0.134783134887   ,  \"σlogτ1\" -> 0.007634654967   ,  \"σlogτS\" -> 0.000261138906   ,  \"σlogτN\" -> 0.003988877910   ,  \"σητ1\" -> 0.004199218371   ,  \"σητS \" -> 0.000025405050   ,  \"σητN\" -> 0.000501380518    |>   , \r\"IDS0599_220609_RAW_cal__sam_\" ->   <|    \"ζ\" -> 0.000000000000   ,  \"τ1\" -> 0.000000000000   ,  \"τS\" -> 0.000000000000   ,  \"τN\" -> 0.000000000000   ,  \"τC\" -> 0.000000000000   ,  \"κ0\" -> 0.000000000000   ,  \"mm1\" -> 0.000000000000   ,  \"mm2\" -> 0.000000000000   ,  \"mm3\" -> 0.000000000000   ,  \"T\" -> 0.250000000000   ,  \"B\" -> 4.000000000000   ,  \"θ\" -> 90.000000000000   ,  \"Reoff\" -> 0.000000000000   ,  \"Imoff\" -> 0.000000000000   ,  \"στ1\" -> 0.000000000000   ,  \"στS\" -> 0.000000000000   ,  \"στN\" -> 0.000000000000   ,  \"τ11 \" -> 0.000000000000   ,  \"τ12\" -> 0.000000000000   ,  \"τ22\" -> 0.000000000000   ,  \"τN1\" -> 0.000000000000   ,  \"τN2\" -> 0.000000000000   ,  \"σηlogτ1 \" -> 0.000000000000   ,  \"σηlogτS\" -> 0.000000000000   ,  \"σηlogτN\" -> 0.000000000000   ,  \"σlogτ1\" -> 0.000000000000   ,  \"σlogτS\" -> 0.000000000000   ,  \"σlogτN\" -> 0.000000000000   ,  \"σητ1\" -> 0.000000000000   ,  \"σητS \" -> 0.000000000000   ,  \"σητN\" -> 0.000000000000    |>   , \r\"IDS0601_220609_RAW_cal__ref_\" ->   <|    \"ζ\" -> 0.076065163691   ,  \"τ1\" -> 0.031218215846   ,  \"τS\" -> 0.032891504670   ,  \"τN\" -> 0.001274630230   ,  \"τC\" -> 0.001592613462   ,  \"κ0\" -> 0.000000001977   ,  \"mm1\" -> 0.000108046468   ,  \"mm2\" -> 0.027306090435   ,  \"mm3\" -> 0.042161679948   ,  \"T\" -> 0.360000000000   ,  \"B\" -> 4.000000000000   ,  \"θ\" -> 90.000000000000   ,  \"Reoff\" -> 0.000000000000   ,  \"Imoff\" -> 0.000000000000   ,  \"στ1\" -> 0.000358946293   ,  \"στS\" -> 0.000004673235   ,  \"στN\" -> 0.000008052665   ,  \"τ11 \" -> 0.000000000000   ,  \"τ12\" -> 0.000000000000   ,  \"τ22\" -> 0.000000000000   ,  \"τN1\" -> 0.000000000000   ,  \"τN2\" -> 0.000000000000   ,  \"σηlogτ1 \" -> 0.120490592225   ,  \"σηlogτS\" -> 0.000188213230   ,  \"σηlogτN\" -> 0.130970976261   ,  \"σlogτ1\" -> 0.011497975887   ,  \"σlogτS\" -> 0.000142080293   ,  \"σlogτN\" -> 0.006317648081   ,  \"σητ1\" -> 0.003761501315   ,  \"σητS \" -> 0.000006190616   ,  \"σητN\" -> 0.000166939566    |>   , \r\"IDS0601_220609_RAW_cal__sam_\" ->   <|    \"ζ\" -> 0.000000000000   ,  \"τ1\" -> 0.000000000000   ,  \"τS\" -> 0.000000000000   ,  \"τN\" -> 0.000000000000   ,  \"τC\" -> 0.000000000000   ,  \"κ0\" -> 0.000000000000   ,  \"mm1\" -> 0.000000000000   ,  \"mm2\" -> 0.000000000000   ,  \"mm3\" -> 0.000000000000   ,  \"T\" -> 0.360000000000   ,  \"B\" -> 4.000000000000   ,  \"θ\" -> 90.000000000000   ,  \"Reoff\" -> 0.000000000000   ,  \"Imoff\" -> 0.000000000000   ,  \"στ1\" -> 0.000000000000   ,  \"στS\" -> 0.000000000000   ,  \"στN\" -> 0.000000000000   ,  \"τ11 \" -> 0.000000000000   ,  \"τ12\" -> 0.000000000000   ,  \"τ22\" -> 0.000000000000   ,  \"τN1\" -> 0.000000000000   ,  \"τN2\" -> 0.000000000000   ,  \"σηlogτ1 \" -> 0.000000000000   ,  \"σηlogτS\" -> 0.000000000000   ,  \"σηlogτN\" -> 0.000000000000   ,  \"σlogτ1\" -> 0.000000000000   ,  \"σlogτS\" -> 0.000000000000   ,  \"σlogτN\" -> 0.000000000000   ,  \"σητ1\" -> 0.000000000000   ,  \"σητS \" -> 0.000000000000   ,  \"σητN\" -> 0.000000000000    |>   , \r\"IDS0602_220609_RAW_cal__ref_\" ->   <|    \"ζ\" -> 0.057533507223   ,  \"τ1\" -> 0.029396748260   ,  \"τS\" -> 0.031273780346   ,  \"τN\" -> 0.000872241596   ,  \"τC\" -> 0.001990785128   ,  \"κ0\" -> 0.000000002387   ,  \"mm1\" -> 0.000102455319   ,  \"mm2\" -> 0.026505841870   ,  \"mm3\" -> 0.038774731527   ,  \"T\" -> 0.420000000000   ,  \"B\" -> 4.000000000000   ,  \"θ\" -> 90.000000000000   ,  \"Reoff\" -> 0.000000000000   ,  \"Imoff\" -> 0.000000000000   ,  \"στ1\" -> 0.000352874051   ,  \"στS\" -> 0.000003364822   ,  \"στN\" -> 0.000005730274   ,  \"τ11 \" -> 0.000000000000   ,  \"τ12\" -> 0.000000000000   ,  \"τ22\" -> 0.000000000000   ,  \"τN1\" -> 0.000000000000   ,  \"τN2\" -> 0.000000000000   ,  \"σηlogτ1 \" -> 0.120950197398   ,  \"σηlogτS\" -> 0.000137548204   ,  \"σηlogτN\" -> 0.130993605381   ,  \"σlogτ1\" -> 0.012003846422   ,  \"σlogτS\" -> 0.000107592440   ,  \"σlogτN\" -> 0.006569595024   ,  \"σητ1\" -> 0.003555542505   ,  \"σητS \" -> 0.000004301652   ,  \"σητN\" -> 0.000114258071    |>   , \r\"IDS0602_220609_RAW_cal__sam_\" ->   <|    \"ζ\" -> 0.000000000000   ,  \"τ1\" -> 0.000000000000   ,  \"τS\" -> 0.000000000000   ,  \"τN\" -> 0.000000000000   ,  \"τC\" -> 0.000000000000   ,  \"κ0\" -> 0.000000000000   ,  \"mm1\" -> 0.000000000000   ,  \"mm2\" -> 0.000000000000   ,  \"mm3\" -> 0.000000000000   ,  \"T\" -> 0.420000000000   ,  \"B\" -> 4.000000000000   ,  \"θ\" -> 90.000000000000   ,  \"Reoff\" -> 0.000000000000   ,  \"Imoff\" -> 0.000000000000   ,  \"στ1\" -> 0.000000000000   ,  \"στS\" -> 0.000000000000   ,  \"στN\" -> 0.000000000000   ,  \"τ11 \" -> 0.000000000000   ,  \"τ12\" -> 0.000000000000   ,  \"τ22\" -> 0.000000000000   ,  \"τN1\" -> 0.000000000000   ,  \"τN2\" -> 0.000000000000   ,  \"σηlogτ1 \" -> 0.000000000000   ,  \"σηlogτS\" -> 0.000000000000   ,  \"σηlogτN\" -> 0.000000000000   ,  \"σlogτ1\" -> 0.000000000000   ,  \"σlogτS\" -> 0.000000000000   ,  \"σlogτN\" -> 0.000000000000   ,  \"σητ1\" -> 0.000000000000   ,  \"σητS \" -> 0.000000000000   ,  \"σητN\" -> 0.000000000000    |>   , \r\"IDS0603_220609_RAW_cal__ref_\" ->   <|    \"ζ\" -> 0.041831727936   ,  \"τ1\" -> 0.022173847352   ,  \"τS\" -> 0.030659717390   ,  \"τN\" -> 0.000376835050   ,  \"τC\" -> 0.002231201000   ,  \"κ0\" -> 0.000000003055   ,  \"mm1\" -> 0.000083944151   ,  \"mm2\" -> 0.021503279099   ,  \"mm3\" -> 0.035152690159   ,  \"T\" -> 0.520000000000   ,  \"B\" -> 4.000000000000   ,  \"θ\" -> 90.000000000000   ,  \"Reoff\" -> 0.000000000000   ,  \"Imoff\" -> 0.000000000000   ,  \"στ1\" -> 0.000311741441   ,  \"στS\" -> 0.000001974777   ,  \"στN\" -> 0.000002711407   ,  \"τ11 \" -> 0.000000000000   ,  \"τ12\" -> 0.000000000000   ,  \"τ22\" -> 0.000000000000   ,  \"τN1\" -> 0.000000000000   ,  \"τN2\" -> 0.000000000000   ,  \"σηlogτ1 \" -> 0.139454796721   ,  \"σηlogτS\" -> 0.000091254795   ,  \"σηlogτN\" -> 0.134491686536   ,  \"σlogτ1\" -> 0.014058969391   ,  \"σlogτS\" -> 0.000064409512   ,  \"σlogτN\" -> 0.007195210096   ,  \"σητ1\" -> 0.003092249375   ,  \"σητS \" -> 0.000002797846   ,  \"σητN\" -> 0.000050681181    |>   , \r\"IDS0603_220609_RAW_cal__sam_\" ->   <|    \"ζ\" -> 0.000000000000   ,  \"τ1\" -> 0.000000000000   ,  \"τS\" -> 0.000000000000   ,  \"τN\" -> 0.000000000000   ,  \"τC\" -> 0.000000000000   ,  \"κ0\" -> 0.000000000000   ,  \"mm1\" -> 0.000000000000   ,  \"mm2\" -> 0.000000000000   ,  \"mm3\" -> 0.000000000000   ,  \"T\" -> 0.520000000000   ,  \"B\" -> 4.000000000000   ,  \"θ\" -> 90.000000000000   ,  \"Reoff\" -> 0.000000000000   ,  \"Imoff\" -> 0.000000000000   ,  \"στ1\" -> 0.000000000000   ,  \"στS\" -> 0.000000000000   ,  \"στN\" -> 0.000000000000   ,  \"τ11 \" -> 0.000000000000   ,  \"τ12\" -> 0.000000000000   ,  \"τ22\" -> 0.000000000000   ,  \"τN1\" -> 0.000000000000   ,  \"τN2\" -> 0.000000000000   ,  \"σηlogτ1 \" -> 0.000000000000   ,  \"σηlogτS\" -> 0.000000000000   ,  \"σηlogτN\" -> 0.000000000000   ,  \"σlogτ1\" -> 0.000000000000   ,  \"σlogτS\" -> 0.000000000000   ,  \"σlogτN\" -> 0.000000000000   ,  \"σητ1\" -> 0.000000000000   ,  \"σητS \" -> 0.000000000000   ,  \"σητN\" -> 0.000000000000    |>   , \r\"IDS0604_220609_RAW_cal__ref_\" ->   <|    \"ζ\" -> 0.032626148375   ,  \"τ1\" -> 0.016295992277   ,  \"τS\" -> 0.030913389463   ,  \"τN\" -> 0.000240237020   ,  \"τC\" -> 0.002587979957   ,  \"κ0\" -> 0.000000003764   ,  \"mm1\" -> 0.000075802373   ,  \"mm2\" -> 0.016078766991   ,  \"mm3\" -> 0.034899452193   ,  \"T\" -> 0.620000000000   ,  \"B\" -> 4.000000000000   ,  \"θ\" -> 90.000000000000   ,  \"Reoff\" -> 0.000000000000   ,  \"Imoff\" -> 0.000000000000   ,  \"στ1\" -> 0.000253503530   ,  \"στS\" -> 0.000001618253   ,  \"στN\" -> 0.000001840465   ,  \"τ11 \" -> 0.000000000000   ,  \"τ12\" -> 0.000000000000   ,  \"τ22\" -> 0.000000000000   ,  \"τN1\" -> 0.000000000000   ,  \"τN2\" -> 0.000000000000   ,  \"σηlogτ1 \" -> 0.168215723146   ,  \"σηlogτS\" -> 0.000092448124   ,  \"σηlogτN\" -> 0.139242705944   ,  \"σlogτ1\" -> 0.015556188633   ,  \"σlogτS\" -> 0.000052347952   ,  \"σlogτN\" -> 0.007661039077   ,  \"σητ1\" -> 0.002741242125   ,  \"σητS \" -> 0.000002857885   ,  \"σητN\" -> 0.000033451253    |>   , \r\"IDS0604_220609_RAW_cal__sam_\" ->   <|    \"ζ\" -> 0.000000000000   ,  \"τ1\" -> 0.000000000000   ,  \"τS\" -> 0.000000000000   ,  \"τN\" -> 0.000000000000   ,  \"τC\" -> 0.000000000000   ,  \"κ0\" -> 0.000000000000   ,  \"mm1\" -> 0.000000000000   ,  \"mm2\" -> 0.000000000000   ,  \"mm3\" -> 0.000000000000   ,  \"T\" -> 0.620000000000   ,  \"B\" -> 4.000000000000   ,  \"θ\" -> 90.000000000000   ,  \"Reoff\" -> 0.000000000000   ,  \"Imoff\" -> 0.000000000000   ,  \"στ1\" -> 0.000000000000   ,  \"στS\" -> 0.000000000000   ,  \"στN\" -> 0.000000000000   ,  \"τ11 \" -> 0.000000000000   ,  \"τ12\" -> 0.000000000000   ,  \"τ22\" -> 0.000000000000   ,  \"τN1\" -> 0.000000000000   ,  \"τN2\" -> 0.000000000000   ,  \"σηlogτ1 \" -> 0.000000000000   ,  \"σηlogτS\" -> 0.000000000000   ,  \"σηlogτN\" -> 0.000000000000   ,  \"σlogτ1\" -> 0.000000000000   ,  \"σlogτS\" -> 0.000000000000   ,  \"σlogτN\" -> 0.000000000000   ,  \"σητ1\" -> 0.000000000000   ,  \"σητS \" -> 0.000000000000   ,  \"σητN\" -> 0.000000000000    |>   , \r\"I
